vi "PlotSelection.vi"() -> (2 "XY Graph":cluster{i32[], i32[]}(graph))   [LabVIEW 2009]
panel:
  out "Selection":T1
  in  "stop":bool
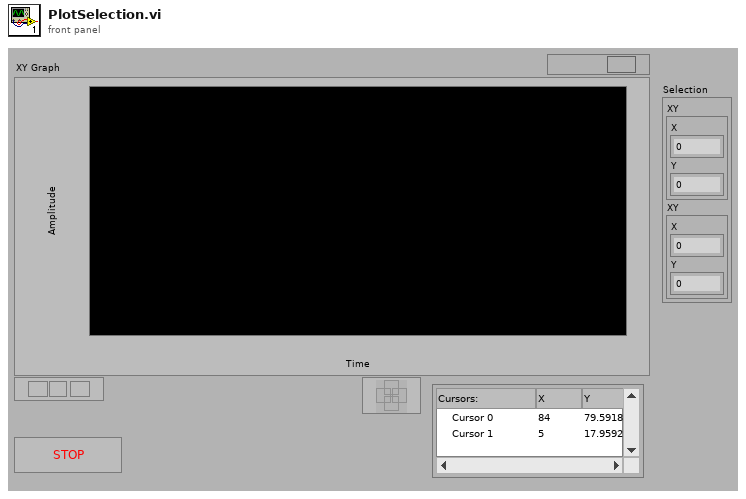
[diagram p1: front panel]
types:
  T1 = cluster{"XY":cluster{"X":dbl, "Y":dbl}, "XY":cluster{"X":dbl, "Y":dbl}}
  T2 = typedef "LVRectTypeDef.ctl" = cluster{"left":i16, "top":i16, "right":i16, "bottom":i16}
  T3 = cluster{"Width":i16, "Style":enum32{"Solid", "Dash", "Dot", "DashDot", "DashDotDot"}}
  T4 = typedef "LVPointDoubleTypeDef.ctl" = cluster{"Cursor X":dbl, "Cursor Y":dbl}
  T5 = typedef "LVPoint32TypeDef.ctl" = cluster{"Horizontal":i32, "Vertical":i32}
  T6 = cluster{"Cursor.Cursor Position":T4, "Cursor.Cursor Position":T4}
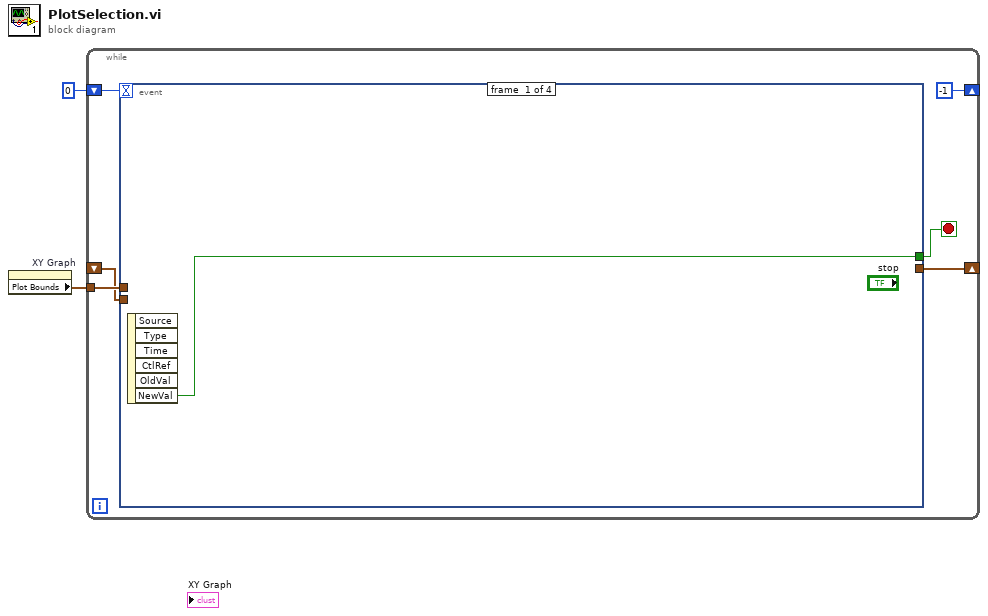
[diagram p0: block diagram]
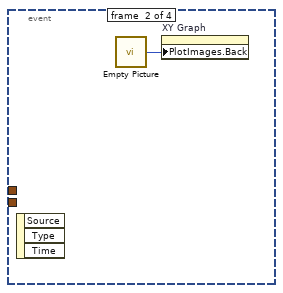
[diagram p2: hidden frame]
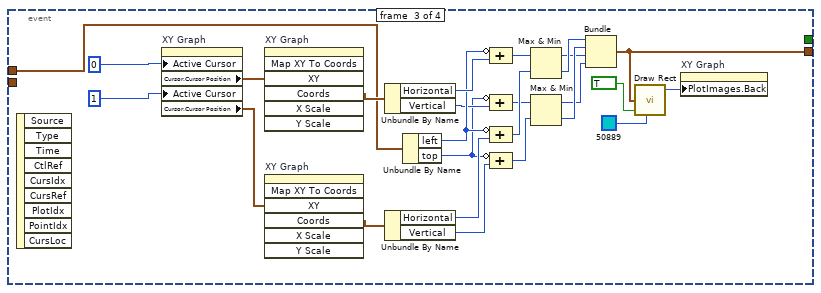
[diagram p3: hidden frame]
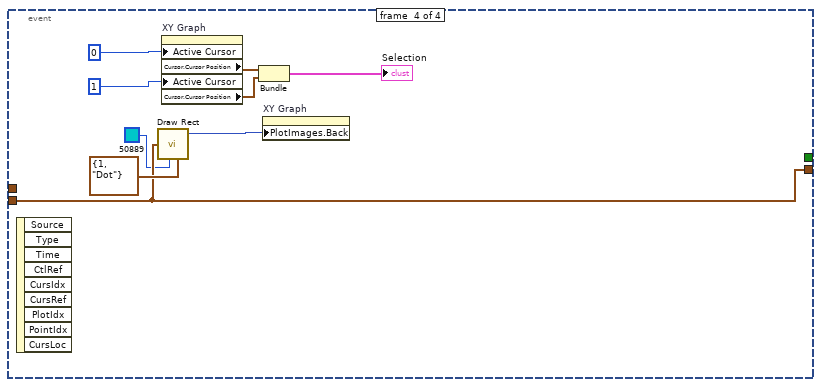
[diagram p4: hidden frame]
diagram:
  n1 = property on="XY Graph" class="XYGraph (strict)"() -> ("Plot Bounds"=w2:T2)  [unwired: 2 in, 2 out]
  n2 = while {
    tunnel: w2 -> [w7]
    shift-right: [w6] -> _
    shift-left: _ -> [w5]
    shift-right: [-1] -> _
    shift-left: 0 -> [w4]
    stop <- w8 stop-if-true
    n3 = event shown="[1] Timeout" {
      selector: _ -> [_ _ _ _]
      dyn-events: _ -> [_ _ _ _]
      timeout: w4 -> [_ _ _ _]
      tunnel: [w9 _ _ _] -> w8
      tunnel: w7 -> [_ _ w23 _]
      tunnel: [_ _ w12 w42] -> w6
      tunnel: w5 -> [_ _ _ w42]
      event #0 {
        n4 = event-data() -> ("NewVal"=w9:bool)  [unwired: 6 out]
      }
      event #1 {
        n5 = event-data() -> ()  [unwired: 4 out]
        n6 = call "Empty Picture"() -> ("empty picture"=w10:picture)
        n7 = property on="XY Graph" class="XYGraph (strict)"("PlotImages.Back"=w10) -> ()  [unwired: 2 in, 2 out]
      }
      event #2 {
        n8 = event-data() -> ()  [unwired: 10 out]
        n9 = property on="XY Graph" class="XYGraph (strict)"("Active Cursor"=u32 0, "Active Cursor"=u32 1) -> ("Cursor.Cursor Position"=w33:T4, "Cursor.Cursor Position"=w32:T4)  [unwired: 2 in, 2 out]
        n10 = invoke on="XY Graph" class="XYGraph (strict)" method="Map XY To Coords"("XY"=w33) -> ("Coords"=w31:T5)  [unwired: 6 in, 6 out]
        n11 = invoke on="XY Graph" class="XYGraph (strict)" method="Map XY To Coords"("XY"=w32) -> ("Coords"=w30:T5)  [unwired: 6 in, 6 out]
        n12 = Unbundle By Name(w31) -> ("Horizontal"=w22:i32, "Vertical"=w17:i32)
        n13 = Unbundle By Name(w30) -> ("Horizontal"=w20:i32, "Vertical"=w15:i32)
        n14 = Unbundle By Name(w23) -> ("left"=w19:i16, "top"=w13:i16)
        n15 = Compound Arithmetic op=ADD(invert w19, w22) -> (w21:i32)
        n16 = Compound Arithmetic op=ADD(invert w13, w17) -> (w16:i32)
        n17 = Compound Arithmetic op=ADD(invert w19, w20) -> (w18:i32)
        n18 = Compound Arithmetic op=ADD(invert w13, w15) -> (w14:i32)
        n19 = Max & Min(x=w21, y=w18) -> (max(x,y)=w26:i32, min(x,y)=w29:i32)
        n20 = Max & Min(x=w16, y=w14) -> (max(x,y)=w27:i32, min(x,y)=w28:i32)
        n21 = Bundle(w29, w28, w26, w27) -> (w12:cluster{i32, i32, i32, i32})  [unwired: 1 out]
        n22 = call <vilib>:"Draw Rect.vi"("rect"=w12, "fill?(F)"=TRUE, "color(black)"=u32 50889) -> ("new picture"=w24:picture)  [unwired: 2 in, 4 out]
        n23 = property on="XY Graph" class="XYGraph (strict)"("PlotImages.Back"=w24) -> ()  [unwired: 2 in, 2 out]
      }
      event #3 {
        n24 = event-data() -> ()  [unwired: 10 out]
        n25 = call <vilib>:"Draw Rect.vi"("rect"=w42, "color(black)"=u32 50889, "pen"=T3 {"Width"=1, "Style"=enum."Dot"}) -> ("new picture"=w44:picture)  [unwired: 2 in, 4 out]
        n26 = property on="XY Graph" class="XYGraph (strict)"("Active Cursor"=u32 0, "Active Cursor"=u32 1) -> ("Cursor.Cursor Position"=w38:T4, "Cursor.Cursor Position"=w37:T4)  [unwired: 2 in, 2 out]
        n27 = Bundle("Cursor.Cursor Position"=w38, "Cursor.Cursor Position"=w37) -> (→"Selection":T6)  [unwired: 1 out]
        n28 = property on="XY Graph" class="XYGraph (strict)"("PlotImages.Back"=w44) -> ()  [unwired: 2 in, 2 out]
      }
    }
  }
